vi "initialize_data_log.vi"(7 "Overwrite?":bool, 8 "error in (no error)":errorcluster, 9 "Initialization Data":variant, 10 "Path":path, 11 "raw_stream_logger in":refnum<class "raw_stream_logger.lvclass">) -> (0 "error out":errorcluster, 3 "raw_stream_logger out":refnum<class "raw_stream_logger.lvclass">)   [LabVIEW 2015, in "raw_stream_logger.lvclass"]
uses:
  raw_stream_logger.lvclass
  raw_stream_logger.lvclass/raw_stream_logger.ctl
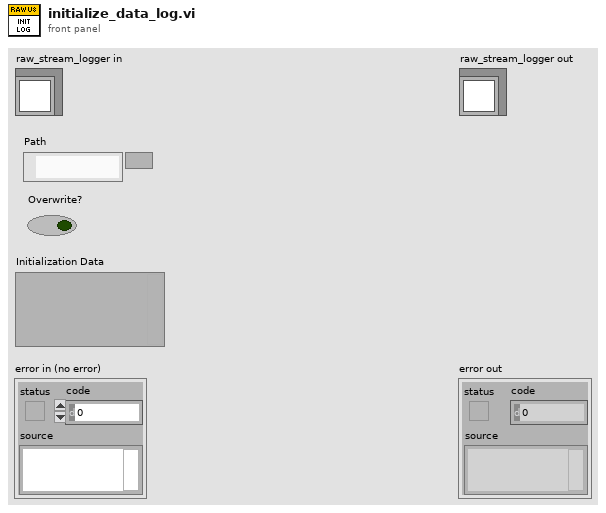
[diagram p1: front panel]
types:
  T1 = enum16{"open", "replace", "create", "open or create", "replace or create", "replace or create with confirmation"}
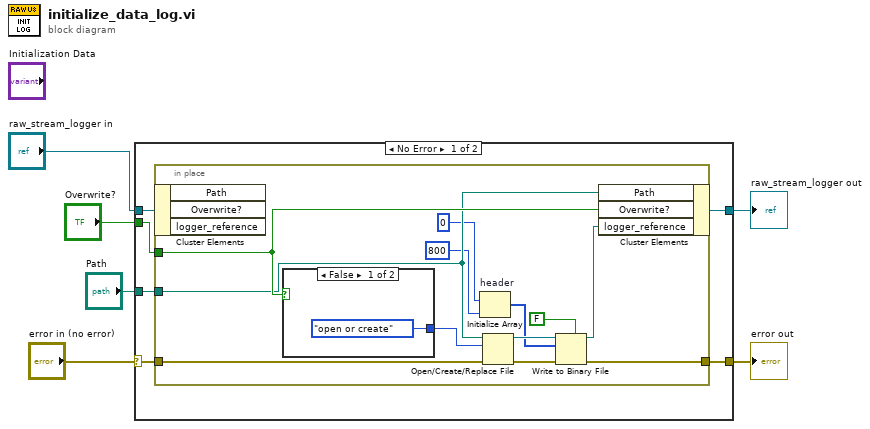
[diagram p0: block diagram]
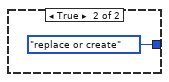
[diagram p2: hidden frame]
diagram:
  n1 = case shown="No Error" "error in (no error)" {
    selector: "error in (no error)" -> [w10 w27]
    tunnel: "Path" -> [w12 _]
    tunnel: "raw_stream_logger in" -> [w11 w28]
    tunnel: [w9 w28] -> w3
    tunnel: "Overwrite?" -> [w8 _]
    tunnel: [w7 w27] -> w1
    frame No Error {
      n2 = in-place {
        in-place-border: w12 -> [w21]
        in-place-border: w10 -> [w24]
        in-place-border: w8 -> [w22]
        in-place-border: [w19] -> w7
        n3 = in-place-cluster #1(w11) -> ()  [unwired: 3 out]
        n4 = case shown="False" w22 {
          tunnel: [T1."open or create" ("operation (0:open)") T1."replace or create" ("operation (0:open)")] -> w23
          frame False {
          }
          frame True {
          }
        }
        n5 = Initialize Array "header"(u8 0, 800 ("dimension size")) -> (w14:u8[])
        n6 = Open/Create/Replace File(file path (use dialog)=w21, error in=w24, operation (0:open)=w23) -> (refnum out=w18:refnum<file>, error out=w20:errorcluster)  [unwired: 3 in, 1 out]
        n7 = Write to Binary File(file (use dialog)=w18, data=w14, error in=w20, 5:FALSE ("prepend array or string size? (T)")) -> (refnum out=w17:refnum<file>, error out=w19:errorcluster)  [unwired: 2 in, 1 out]
        n8 = in-place-cluster #1("Path"=w21, "Overwrite?"=w22, "logger_reference"=w17) -> (w9:refnum<class "raw_stream_logger.lvclass">)
      }
    }
    frame Error {
    }
  }
  "error out" <- w1
  "raw_stream_logger out" <- w3
